vi "Korona2012.vi"() -> ()   [LabVIEW 2010]
uses:
  <instrlib>/niScope/Controls/niScope vertical coupling.ctl
  <instrlib>/niScope/Controls/niScope trigger coupling.ctl
  <instrlib>/niScope/Controls/niScope trigger slope.ctl
  <instrlib>/niScope/Controls/niScope trigger source.ctl
  <instrlib>/niSync/niSync.llb/niSync Initialize (IVI).vi
  <instrlib>/niSync/niSync.llb/niSync Set Time Reference (GPS).vi
  <instrlib>/niScope/Configure/Trigger/niScope Configure Trigger Edge.vi
  <instrlib>/niScope/Acquire/Fetch/niScope Multi Fetch Binary 16.vi
  <instrlib>/niSync/niSync.llb/niSync Read Trigger Time Stamp (Multiple).vi
panel:
  out "Num":i32
  out "# elements in queue":i32
  out "etime":dbl format="%<%H:%M:%S%1u>t"
  in  "Numeric":i32=32
  out "GPS:Status":i32(ring) items=["Uninitialized", "Antenna Error", "No Useable Satellites", "One Useable Satellite", "Two Useable Satellites", "Three Useable Satellites", "No GPS Time", "PDOP Too High", "Unuseable Satellite", "Fix Rejected", "Self Survey Complete", "Self Survey Not Complete"]
  out "Device:Temperature":dbl
  out "error out":errorcluster
  # "Скорость записи на диск ~20МБ/с.\nКаждая запись тоже ~20МБ, \nбез буферизации - одна запись/с.\nСовместно с очередью на 20 элементов\nуспеваем зарегистрировать 32 записи на 10с."
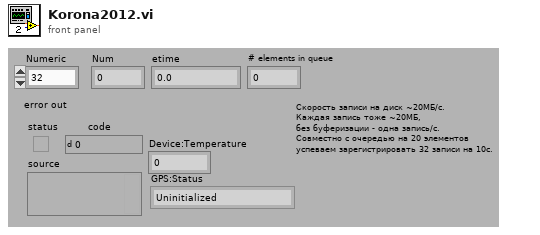
[diagram p1: front panel]
types:
  T1 = cluster{cluster{"actualSamples":i32, "absoluteInitialX":dbl, "relativeInitialX":dbl, "xIncrement":dbl, "offset":dbl, "gain":dbl, "reserved1":dbl, "reserved2":dbl}[], "wfm":i16[][]}
  T2 = typedef "niScope trigger source.ctl" = string
  T3 = typedef "niScope trigger slope.ctl" = i32
  T4 = typedef "niScope trigger coupling.ctl" = u16
  T5 = typedef "niScope vertical coupling.ctl" = i32
  T6 = cluster{"actualSamples":i32, "absoluteInitialX":dbl, "relativeInitialX":dbl, "xIncrement":dbl, "offset":dbl, "gain":dbl, "reserved1":dbl, "reserved2":dbl}[]
  T7 = cluster{"actualSamples":i32, "absoluteInitialX":dbl, "relativeInitialX":dbl, "xIncrement":dbl, "offset":dbl, "gain":dbl, "reserved1":dbl, "reserved2":dbl}
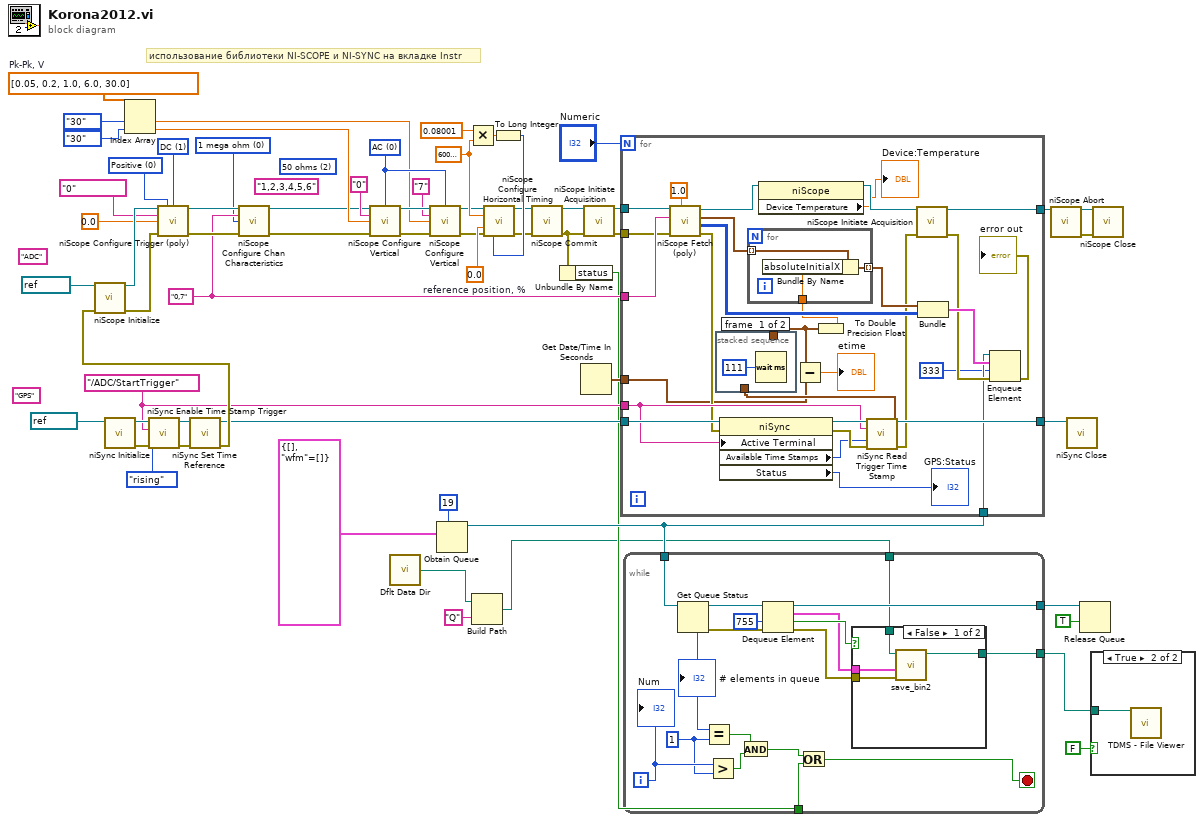
[diagram p0: block diagram]
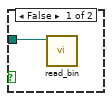
[diagram p3: hidden frame]
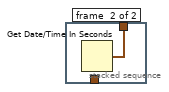
[diagram p4: hidden frame]
diagram:
  (unwired) u32 2 items=["1 mega ohm"=0, "50 ohms"=2] ("input impedance")
  (unwired) "1,2,3,4,5,6" ("channels")
  w36 = tag "/ADC/StartTrigger" ("terminal")
  w55 = dbl[] [0.05, 0.2, 1.0, 6.0, 30.0]  # Pk-Pk, V
  w47 = T3 0 items=["Positive", "Negative"] ("trigger slope")
  w48 = T4 1 items=["AC"=0, "DC"=1, "HF Reject"=3, "LF Reject"=4, "AC Plus HF Reject"=1001] ("trigger coupling")
  w56 = u32 0 items=["1 mega ohm"=0, "50 ohms"=2] ("input impedance")
  w52 = 60000000.0 ("min sample rate")
  w61 = 0.0  # reference position, %
  w22 = T5 0 items=["AC", "DC", "Ground"] ("vertical coupling")
  w57 = "0,7" ("channels")
  (unwired) "GPS"
  (unwired) "ADC"
  # "использование библиотеки NI-SCOPE и NI-SYNC на вкладке Instr"
  n1 = call-poly <instrlib>:"niSync Initialize.vi"("resource name"=refnum<k15> "GPS") -> ("error out"=w44:errorcluster, "instrument handle out"=w38:refnum<k15>)  [unwired: 9 in]
  n2 = Index Array(array=w55, index #1=enum16{"1/20", "1/5", "1", "6", "30"}."30", index #2=enum16{"1/20", "1/5", "1", "6", "30"}."30") -> (element #1=w21:dbl, element #2=w20:dbl)
  n3 = call <instrlib>:"niSync Enable Time Stamp Trigger.vi"("error in (no error)"=w44, "active edge"=enum32{"rising", "falling", "any"}."rising", "terminal"=w36, "instrument handle"=w38) -> ("error out"=w41:errorcluster, "instrument handle out"=w42:refnum<k15>)  [unwired: 5 in]
  n4 = call-poly <instrlib>:"niSync Set Time Reference.vi"("error in (no error)"=w41, "instrument handle"=w42) -> ("error out"=w37:errorcluster, "instrument handle out"=w33:refnum<k15>)  [unwired: 8 in]
  n5 = call <instrlib>:"niScope Initialize.vi"("resource name"=refnum<k15> "ADC", "error in"=w37) -> ("instrument handle"=w62:refnum<k15>, "error out"=w60:errorcluster)  [unwired: 12 in]
  n6 = call-poly <instrlib>:"niScope Configure Trigger (poly).vi"("instrument handle"=w62, "trigger slope"=w47, "trigger coupling"=w48, "trigger source"=T2 "0", "trigger level"=0.0, "error in"=w60) -> ("instrument handle out"=w59:refnum<k15>, "error out"=w58:errorcluster)  [unwired: 8 in]
  n7 = call <instrlib>:"niScope Configure Chan Characteristics.vi"("instrument handle"=w59, "channels"=w57, "input impedance"=w56, "error in"=w58) -> ("instrument handle out"=w18:refnum<k15>, "error out"=w17:errorcluster)  [unwired: 10 in]
  n8 = call <instrlib>:"niScope Configure Vertical.vi"("instrument handle"=w18, "vertical coupling"=w22, "channels"="0", "vertical range"=w20, "error in"=w17) -> ("instrument handle out"=w25:refnum<k15>, "error out"=w26:errorcluster)  [unwired: 9 in]
  n9 = call <vilib>:"Dflt Data Dir.vi"() -> ("App:Default Data Directory"=w3:path)
  n10 = call <instrlib>:"niScope Configure Vertical.vi"("instrument handle"=w25, "vertical coupling"=w22, "channels"="7", "vertical range"=w21, "error in"=w26) -> ("instrument handle out"=w23:refnum<k15>, "error out"=w24:errorcluster)  [unwired: 9 in]
  n11 = Obtain Queue(max queue size (-1, unlimited)=19, element data type=T1 {[], "wfm"=[]} ("output cluster")) -> (queue out=w9:refnum<queue>)  [unwired: 3 in, 2 out]
  n12 = Multiply(x=0.08001, y=w52) -> (x*y=w50:dbl)
  n13 = Build Path(base path=w3, name or relative path="Q") -> (appended path=w1:path)
  n14 = To Long Integer(number=w50) -> (32bit integer=w49:i32)
  n15 = call <instrlib>:"niScope Configure Horizontal Timing.vi"("instrument handle"=w23, "min sample rate"=w52, "reference position"=w61, "error in"=w24, "min record length"=w49) -> ("instrument handle out"=w29:refnum<k15>, "error out"=w30:errorcluster)  [unwired: 9 in]
  n16 = call <instrlib>:"niScope Commit.vi"("instrument handle"=w29, "error in"=w30) -> ("instrument handle out"=w53:refnum<k15>, "error out"=w6:errorcluster)  [unwired: 12 in]
  n17 = Unbundle By Name(w6) -> ("status"=w5:bool)
  n18 = Get Date/Time In Seconds() -> (seconds since 1Jan1904=w15:timestamp)
  n19 = call <instrlib>:"niScope Initiate Acquisition.vi"("instrument handle"=w53, "error in"=w6) -> ("instrument handle out"=w39:refnum<k15>, "error out"=w40:errorcluster)  [unwired: 12 in]
  n20 = for {
    N: "Numeric" -> [_]
    tunnel: w57 -> [w92]
    tunnel: w40 -> [w91]
    tunnel: w39 -> [w90]
    tunnel: [w86] -> w14
    tunnel: w33 -> [w84]
    tunnel: w36 -> [w81]
    tunnel: [w79] -> w35
    tunnel: w15 -> [w74]
    tunnel: w9 -> [w65]
    n21 = call-poly <instrlib>:"niScope Fetch (poly).vi"("timeout"=1.0, "error in"=w91, "channels"=w92, "instrument handle"=w90) -> ("error out"=w80:errorcluster, "wfm"=w89:i16[][], "wfm info"=w88:T6, "instrument handle out"=w70:refnum<k15>)  [unwired: 4 in]
    n22 = property class="niSync"(reference=w84, error in=w80, "Active Terminal"=w81) -> (reference out=w83:refnum<k15>, error out=w85:errorcluster, "Available Time Stamps"=w82:i32, "Status"=→"GPS:Status":i32)
    n23 = property class="niScope"(reference=w70) -> (reference out=w69:refnum<k15>, "Device Temperature"=→"Device:Temperature":dbl)  [unwired: 1 in, 1 out]
    n24 = call-poly <instrlib>:"niSync Read Trigger Time Stamp.vi"("instrument handle"=w83, "terminal"=w81, "number of timestamps"=w82, "error in (no error)"=w85) -> ("instrument handle out"=w86:refnum<k15>, "time stamp out"=w76:timestamp[], "error out"=w77:errorcluster)  [unwired: 8 in, 1 out]
    n25 = stacked-sequence {
      tunnel: w76 -> [_ _]
      tunnel: [_ w94] -> w72
      frame #0 {
        n26 = Wait (ms)(milliseconds to wait=u32 111) -> ()  [unwired: 1 out]
      }
      frame #1 {
        n27 = Get Date/Time In Seconds() -> (seconds since 1Jan1904=w94:timestamp)
      }
    }
    n28 = Subtract(x=w72, y=w74) -> (x-y=→"etime":dbl)
    n29 = To Double Precision Float(number=w72) -> (double precision float=w75:dbl)
    n30 = for {
      tunnel: w88 -> [w97] mode=indexing
      tunnel: w75 -> [w96]
      tunnel: [w95] -> w87 mode=indexing
      n31 = Bundle By Name(cluster=w97, "absoluteInitialX"=w96) -> (w95:T7)
    }
    n32 = call <instrlib>:"niScope Initiate Acquisition.vi"("instrument handle"=w69, "error in"=w77) -> ("instrument handle out"=w79:refnum<k15>, "error out"=w66:errorcluster)  [unwired: 12 in]
    n33 = Bundle(w87, "wfm"=w89) -> (w67:T1)  [unwired: 1 in]
    n34 = Enqueue Element(queue=w65, element=w67, timeout in ms (-1)=333, error in (no error)=w66) -> (error out=→"error out":errorcluster)  [unwired: 2 out]
  }
  n35 = while {
    tunnel: w9 -> [w115]
    tunnel: [w111] -> w8
    tunnel: w1 -> [w109]
    tunnel: w5 -> [w106]
    tunnel: [w104] -> w4
    i -> [w100]
    stop <- w105 stop-if-true
    w98 = 1 ("x")
    n36 = Get Queue Status(queue=w115) -> (queue out=w114:refnum<queue>, error out=w113:errorcluster, # elements in queue=w101:i32)  [unwired: 2 in, 5 out]
    "# elements in queue" <- w101
    n37 = Equal?(x=w101, y=w98) -> (x = y?=w102:bool)
    n38 = Greater?(x=w100, y=w98) -> (0:w99:bool)
    n39 = And(x=w102, y=w99) -> (x .and. y?=w107:bool)
    n40 = Dequeue Element(queue=w114, timeout in ms (-1)=755, error in (no error)=w113) -> (queue out=w111:refnum<queue>, element=w103:T1, timed out?=w110:bool, error out=w112:errorcluster)
    n41 = Or(x=w107, y=w106) -> (x .or. y?=w105:bool)
    n42 = case shown="False" w110 {
      tunnel: w112 -> [w119 _]
      tunnel: w103 -> [w118 _]
      tunnel: w109 -> [w117 _]
      tunnel: [w116 _] -> w104
      frame False {
        n43 = call "save_bin2.vi"("error in"=w119, "xz"=w118, "start path"=w117) -> ("file path out"=w116:path)  [unwired: 2 in, 2 out]
      }
      frame True {
      }
    }
    "Num" <- w100
  }
  n44 = call <instrlib>:"niScope Abort.vi"("instrument handle"=w35) -> ("instrument handle out"=w12:refnum<k15>, "error out"=w13:errorcluster)  [unwired: 13 in]
  n45 = call <instrlib>:"niSync Close.vi"("instrument handle"=w14) -> ()  [unwired: 10 in, 1 out]
  n46 = Release Queue(queue=w8, force destroy? (F)=TRUE) -> ()  [unwired: 1 in, 3 out]
  n47 = case shown="True" FALSE {
    tunnel: w4 -> [w120 w121]
    frame False {
      n48 = call "read_bin.vi"("datalog path"=w120) -> ()  [unwired: 3 in, 4 out]
    }
    frame True {
      n49 = call <vilib>:"TDMS - File Viewer.vi"("file path"=w121) -> ()  [unwired: 5 in, 2 out]
    }
  }
  n50 = call <instrlib>:"niScope Close.vi"("instrument handle"=w12, "error in"=w13) -> ()  [unwired: 13 in, 1 out]
